vi "slope_to_flow.vi"(9 "slope":dbl, 10 "Sampling Frequency [Hz]":dbl, 11 "L/pulse":dbl) -> (3 "Flow [L/min]":dbl)   [LabVIEW 2025, in "LabJackEKG.lvlib"]
uses:
  LabJackEKG.lvlib
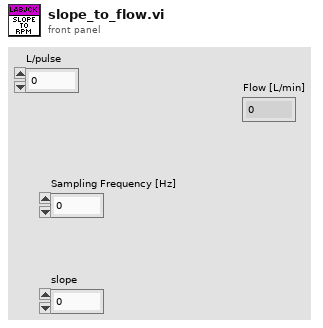
[diagram p1: front panel]
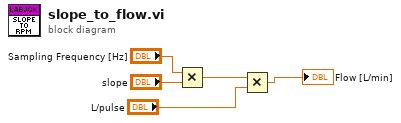
[diagram p0: block diagram]
diagram:
  n1 = Multiply(x="Sampling Frequency [Hz]", y="slope") -> (x*y=w3:dbl)
  n2 = Multiply(x=w3, y="L/pulse") -> (x*y=→"Flow [L/min]":dbl)
